vi "Error Query.vi"(8 "error in (no error)":errorcluster, 11 "VISA resource name":refnum<visa-resource-name>) -> (0 "error out":errorcluster, 1 "String":string caption="Error Message", 2 "Error Code":i32[](array[numeric]), 3 "VISA resource name output":refnum<visa-resource-name>)   [LabVIEW 2018, in "Keithley 3706.lvlib"]
uses:
  <instrlib>/Keithley 3706/Keithley 3706.lvlib
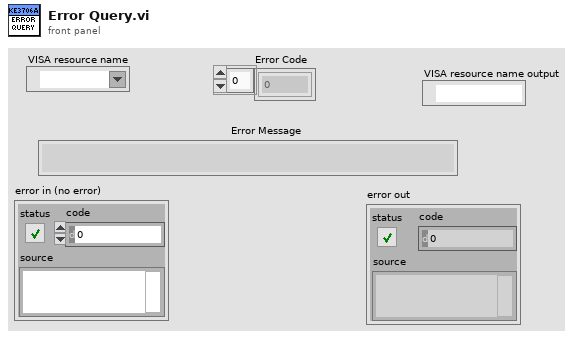
[diagram p1: front panel]
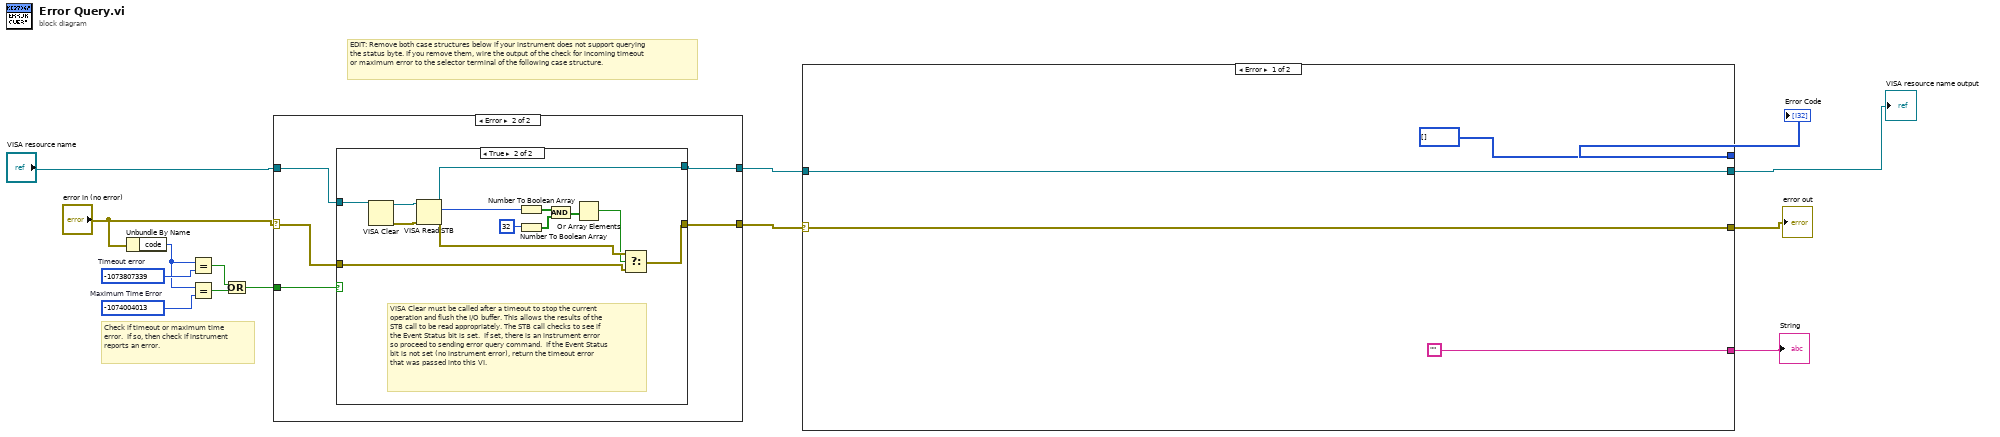
[diagram p0: block diagram]
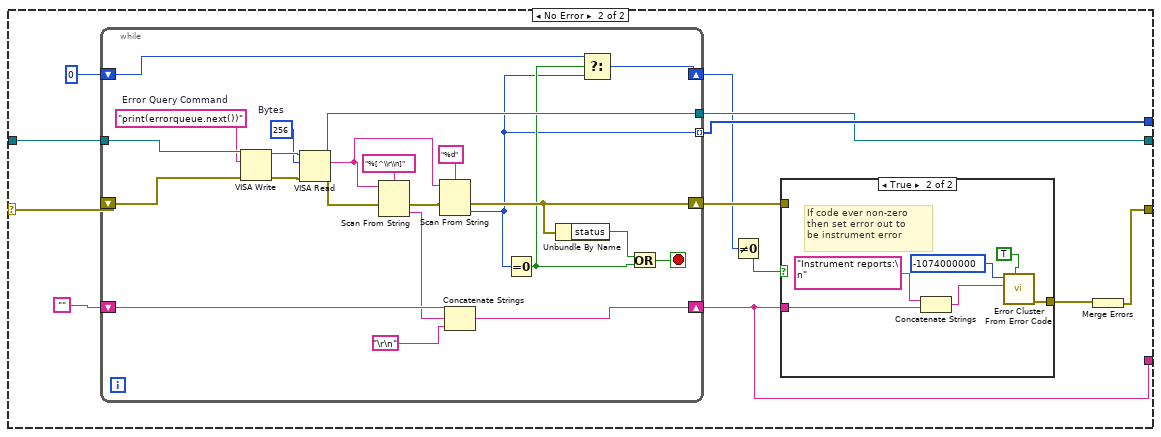
[diagram p2: hidden frame]
diagram:
  w12 = -1074004013  # Maximum Time Error
  w14 = -1073807339  # Timeout error
  # "Check if timeout or maximum time error.  If so, then check if instrument reports an error."
  # "EDIT: Remove both case structures below if your instrument does not support querying the status byte. If you remove them, wire the output of the check for incoming timeout or maximum error to the selector terminal of the following case structure."
  n1 = Unbundle By Name("error in (no error)") -> ("code"=w13:i32)
  n2 = Equal?(x=w13, y=w14) -> (x = y?=w10:bool)
  n3 = Equal?(x=w13, y=w12) -> (x = y?=w11:bool)
  n4 = Or(x=w10, y=w11) -> (x .or. y?=w8:bool)
  n5 = case shown="Error" "error in (no error)" {
    selector: "error in (no error)" -> [w15 w20]
    tunnel: "VISA resource name" -> [w16 w21]
    tunnel: [w16 w18] -> w6
    tunnel: [w15 w17] -> w7
    tunnel: w8 -> [_ w19]
    frame No Error {
    }
    frame Error {
      n6 = case shown="True" w19 {
        tunnel: w21 -> [w23 w36]
        tunnel: [w23 w33] -> w18
        tunnel: w20 -> [w22 w25]
        tunnel: [w22 w24] -> w17
        frame False {
          # "Error code not a timeout, so best to pass on to user."
        }
        frame True {
          # "VISA Clear must be called after a timeout to stop the current operation and flush the I/O buffer. This allows the results of the  STB call to be read appropriately. The STB call checks to see if the Event Status bit is set.  If set, there is an instrument error so proceed to sending error query command.  If the Event Status bit is not set (no instrument error), return the timeout error that was passed into this VI."
          n7 = VISA Clear(VISA resource name=w36) -> (VISA resource name out=w35:refnum<visa-resource-name>, error out=w34:errorcluster)  [unwired: 1 in]
          n8 = VISA Read STB(8:w34, 11:w35) -> (0:w27:errorcluster, 2:w28:u16, 3:w33:refnum<visa-resource-name>)
          n9 = Number To Boolean Array(number=w28) -> (Boolean array=w32:bool[])
          n10 = Number To Boolean Array(number=32) -> (Boolean array=w30:bool[])
          n11 = And(x=w32, y=w30) -> (x .and. y?=w31:bool[])
          n12 = Or Array Elements(Boolean array=w31) -> (logical OR=w26:bool)
          n13 = Select(t=w27, s=w26, f=w25) -> (s? t:f=w24:errorcluster)
        }
      }
    }
  }
  n14 = case shown="Error" w7 {
    selector: w7 -> [w39 w49]
    tunnel: w6 -> [w40 w52]
    tunnel: [w40 w47] -> w1
    tunnel: [w39 w41] -> w5
    tunnel: [i32[] [] w48] -> w3
    tunnel: ["" w45] -> w4
    frame Error {
    }
    frame No Error {
      n15 = while {
        tunnel: w52 -> [w82]
        shift-right: [w66] -> w46
        shift-left: w49 -> [w81]
        shift-right: [w68] -> w45
        shift-left: "" -> [w70]
        shift-right: [w61] -> w44
        shift-left: 0 -> [w63]
        tunnel: [w76] -> w47
        tunnel: [w60] -> w48 mode=indexing
        stop <- w64 stop-if-true
        w77 = u32 256  # Bytes
        w80 = "print(errorqueue.next())"  # Error Query Command
        n16 = VISA Write(VISA resource name=w82, write buffer=w80, error in (no error)=w81) -> (VISA resource name out=w79:refnum<visa-resource-name>, error out=w78:errorcluster)  [unwired: 1 out]
        n17 = VISA Read(VISA resource name=w79, byte count=w77, error in (no error)=w78) -> (VISA resource name out=w76:refnum<visa-resource-name>, read buffer=w73:string, error out=w74:errorcluster)  [unwired: 1 out]
        n18 = Scan From String(format string="%[^\\r\\n]", input string=w73, error in=w74) -> (error out=w72:errorcluster, output 1=w69:string)  [unwired: 2 in, 2 out]
        n19 = Scan From String(format string="%d", input string=w73, error in=w72) -> (error out=w66:errorcluster, output 1=w60:i32)  [unwired: 2 in, 2 out]
        n20 = Concatenate Strings(w70, w69, "\r\n") -> (w68:string)
        n21 = Equal To 0?(x=w60) -> (x = 0?=w62:bool)
        n22 = Unbundle By Name(w66) -> ("status"=w65:bool)
        n23 = Select(t=w63, s=w62, f=w60) -> (s? t:f=w61:i32)
        n24 = Or(x=w65, y=w62) -> (x .or. y?=w64:bool)
      }
      n25 = Not Equal To 0?(x=w44) -> (x != 0?=w43:bool)
      n26 = case shown="True" w43 {
        tunnel: w46 -> [w53 _]
        tunnel: w45 -> [_ w59]
        tunnel: [w53 w54] -> w42
        frame False {
        }
        frame True {
          # "If code ever non-zero\nthen set error out to\nbe instrument error"
          n27 = Concatenate Strings("Instrument reports:\n" ("Source"), w59) -> (w57:string)
          n28 = call <vilib>:"Error Cluster From Error Code.vi"("show call chain? (False)"=TRUE, "error message (\"\")"=w57, "error code (0)"=-1074000000 ("Code")) -> ("error out"=w54:errorcluster)  [unwired: 6 in]
        }
      }
      n29 = Merge Errors(w42) -> (w41:errorcluster)
    }
  }
  "error out" <- w5
  "String" <- w4
  "Error Code" <- w3
  "VISA resource name output" <- w1
